vi "_builtins_rename_label.vi"(8 "error in (no error)":errorcluster, 10 "Label":string, 11 "GObject in":refnum<vi>) -> (0 "error out":errorcluster, 2 "has label?":bool, 3 "GObject out":refnum<vi>)   [LabVIEW 2019, in "Script.lvlib"]
doc: "Renames the GObject label if exists and moves the label to the appropriate position. If the label is empty this does nothing.\n\nCreated by: Ryan Pacini"
uses:
  _builtins_label_position.ctl
  Script.lvlib
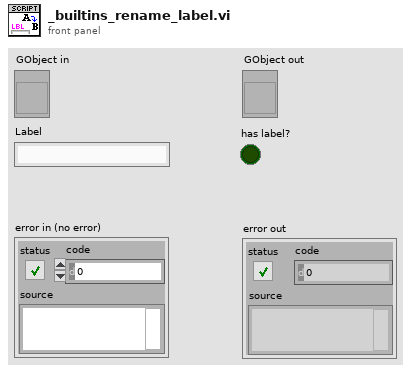
[diagram p1: front panel]
types:
  T1 = typedef "Script.lvlib/_builtins_label_position.ctl" = enum8{"Unchanged", "Top-left", "Top-middle", "Top-right", "Right-top", "Right-middle", "Right-bottom", "Bottom-right", "Bottom-middle", "Bottom-left", "Left-bottom", "Left-middle", "Left-top"}
  T2 = typedef "LVRectTypeDef.ctl" = cluster{"Left":i16, "Top":i16, "Right":i16, "Bottom":i16}
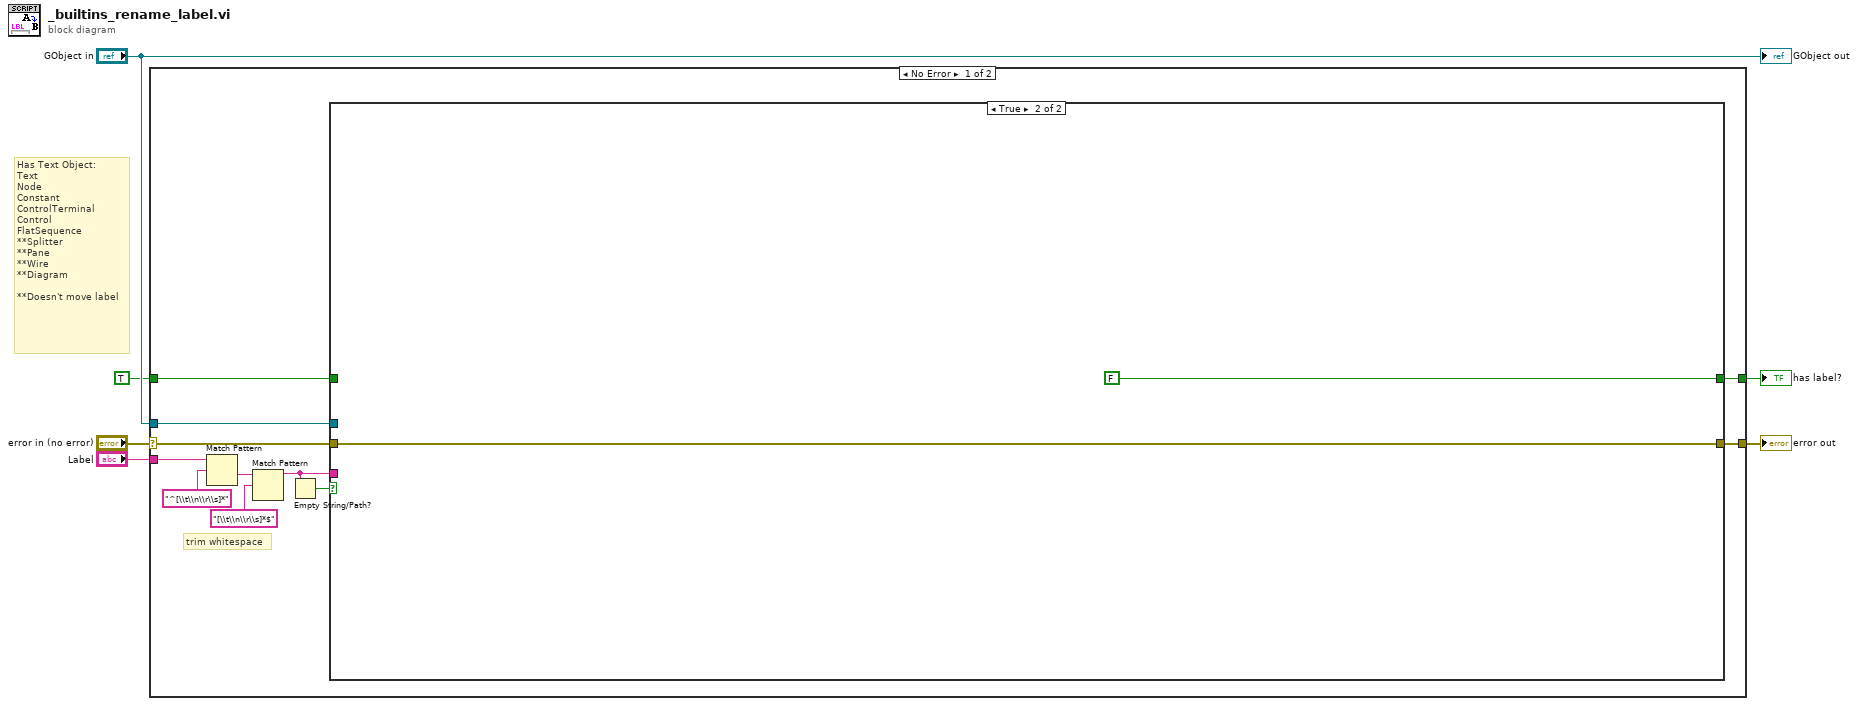
[diagram p0: block diagram]
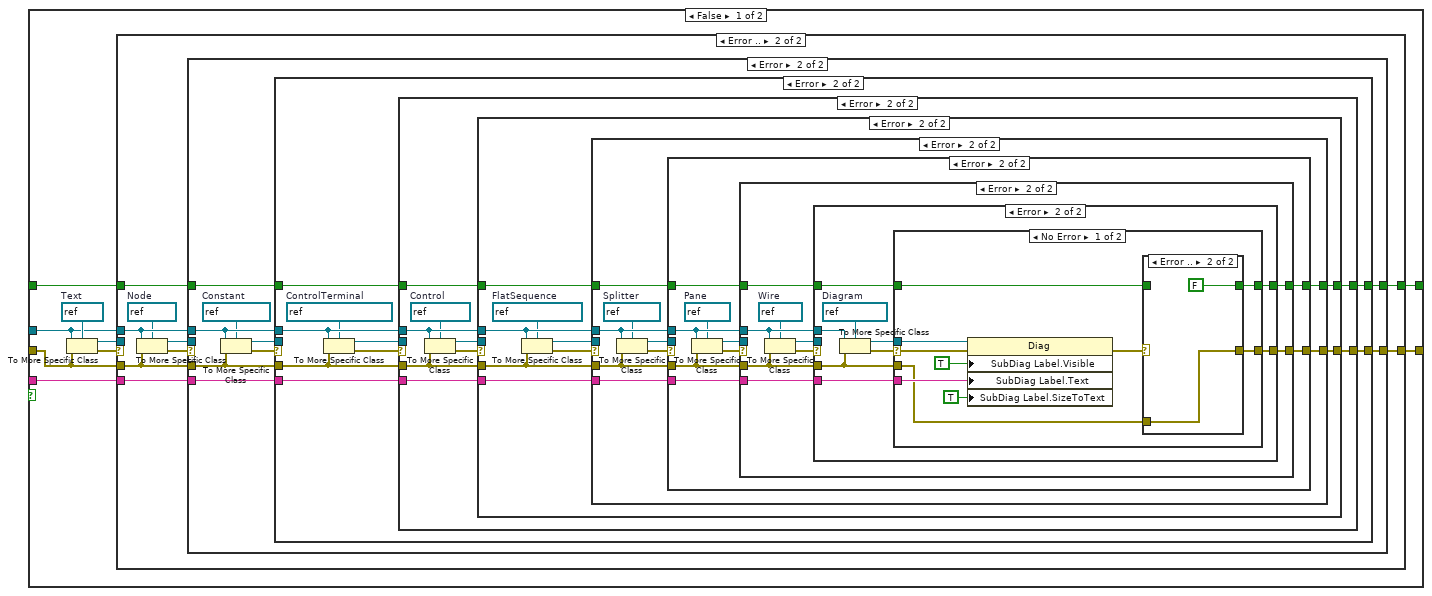
[diagram p2: hidden frame]
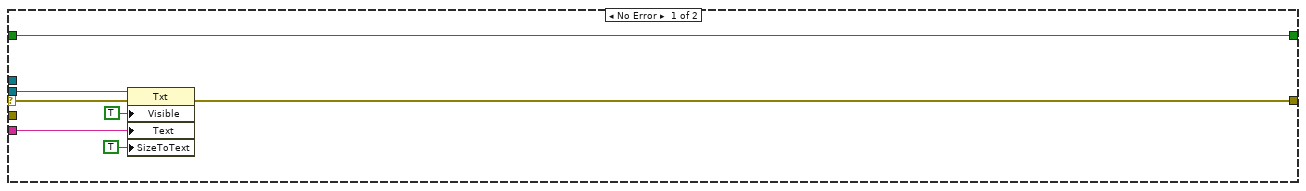
[diagram p3: hidden frame]
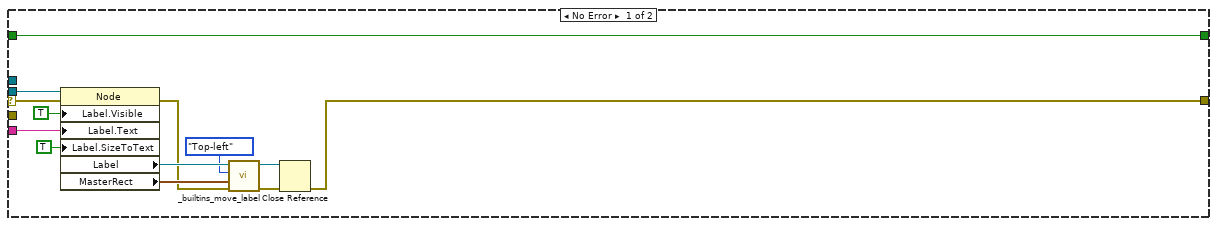
[diagram p4: hidden frame]
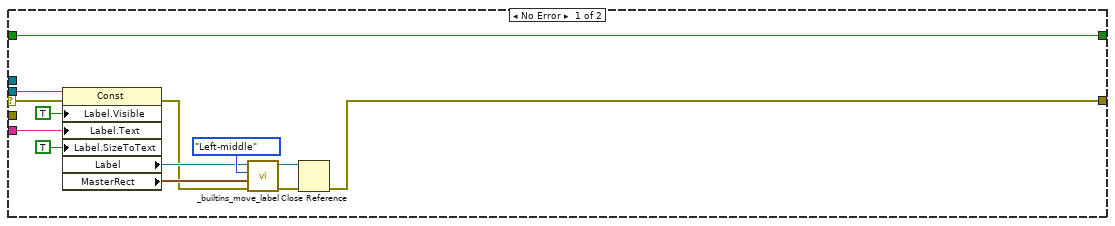
[diagram p5: hidden frame]
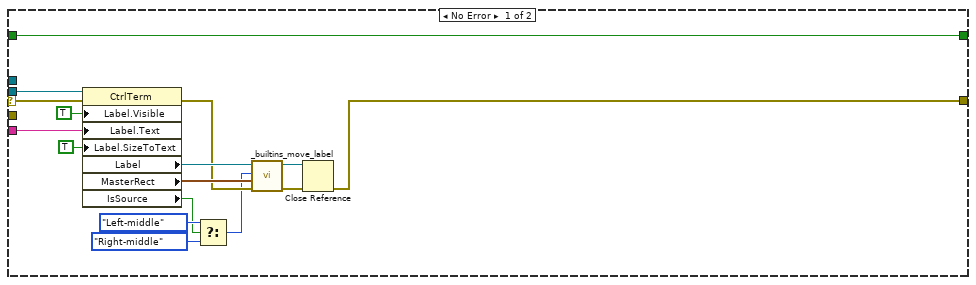
[diagram p6: hidden frame]
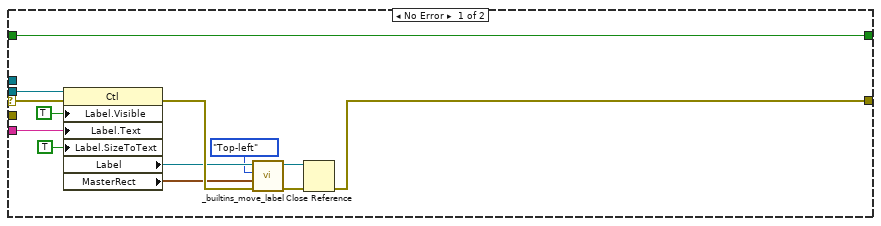
[diagram p7: hidden frame]
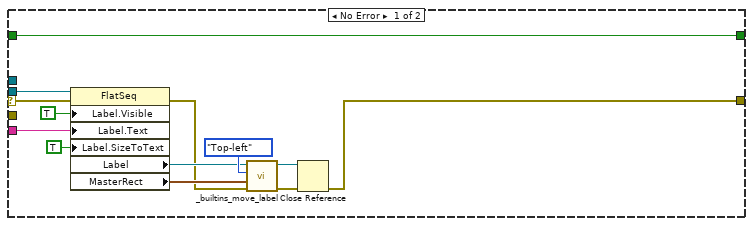
[diagram p8: hidden frame]
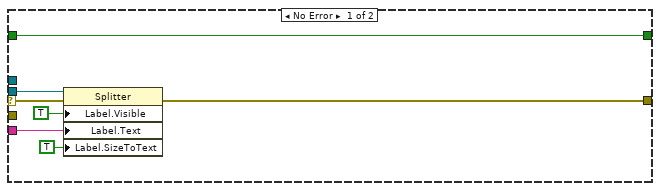
[diagram p9: hidden frame]
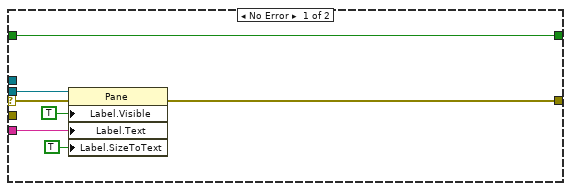
[diagram p10: hidden frame]
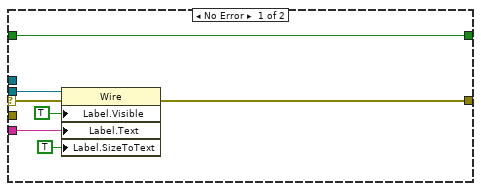
[diagram p11: hidden frame]
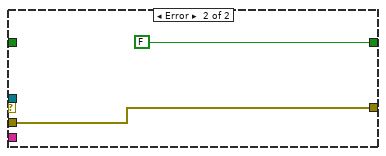
[diagram p13: hidden frame]
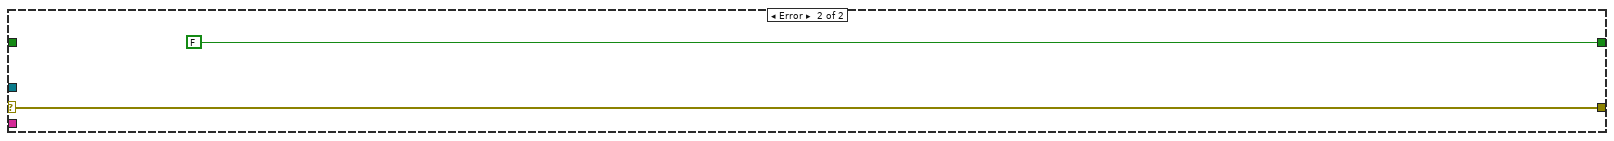
[diagram p14: hidden frame]
diagram:
  # "Has Text Object:\nText\nNode\nConstant\nControlTerminal\nControl\nFlatSequence\n**Splitter\n**Pane\n**Wire\n**Diagram\n\n**Doesn't move label"
  n1 = case shown="No Error" "error in (no error)" {
    selector: "error in (no error)" -> [w14 w223]
    tunnel: "GObject in" -> [w13 _]
    tunnel: [w17 w223] -> w2
    tunnel: [w16 FALSE] -> w3
    tunnel: "Label" -> [w9 _]
    tunnel: TRUE -> [w15 _]
    frame No Error {
      # "trim whitespace"
      n2 = Match Pattern(string=w9, regular expression="^[\\t\\n\\r\\s]*") -> (after substring=w12:string)  [unwired: 1 in, 3 out]
      n3 = Match Pattern(string=w12, regular expression="[\\t\\n\\r\\s]*$") -> (before substring=w8:string)  [unwired: 1 in, 3 out]
      n4 = Empty String/Path?(string/path=w8) -> (empty?=w7:bool)
      n5 = case shown="True" w7 {
        tunnel: [w26 w220] -> w17
        tunnel: [w25 FALSE] -> w16
        tunnel: w8 -> [w24 _]
        tunnel: w15 -> [w23 _]
        tunnel: w14 -> [w21 w220]
        tunnel: w13 -> [w20 _]
        frame False {
          w22 = refnum<vi> refnum  # Text
          n6 = To More Specific Class(target class=w22, reference=w20, error in=w21) -> (specific class reference=w18:refnum<vi>, error out=w19:errorcluster)
          n7 = case shown="Error .." w19 {
            selector: w19 -> [w32 _]
            tunnel: [w29 w42] -> w26
            tunnel: [w28 w41] -> w25
            tunnel: w21 -> [_ w38]
            tunnel: w20 -> [_ w37]
            tunnel: w24 -> [w31 w35]
            tunnel: w23 -> [w28 w34]
            tunnel: w18 -> [w33 _]
            frame No Error {
              n8 = property class="Txt"(reference=w33, error in=w32, "Visible"=TRUE, "Text"=w31, "SizeToText"=TRUE ("Size to Text?")) -> (error out=w29:errorcluster)  [unwired: 1 out]
            }
            frame Error {
              w36 = refnum<vi> refnum  # Node
              n9 = To More Specific Class(target class=w36, reference=w37, error in=w38) -> (specific class reference=w39:refnum<vi>, error out=w40:errorcluster)
              n10 = case shown="Error" w40 {
                selector: w40 -> [w55 _]
                tunnel: w37 -> [_ w62]
                tunnel: w39 -> [w54 _]
                tunnel: w38 -> [_ w61]
                tunnel: [w51 w60] -> w41
                tunnel: [w44 w59] -> w42
                tunnel: w35 -> [w52 w57]
                tunnel: w34 -> [w51 w56]
                frame No Error {
                  n11 = property class="Node"(reference=w54, error in=w55, "Label.Visible"=TRUE, "Label.Text"=w52, "Label.SizeToText"=TRUE ("Label.Size to Text?")) -> (error out=w45:errorcluster, "Label"=w50:refnum<vi>, "MasterRect"=w49:T2)  [unwired: 1 out]
                  n12 = call "_builtins_move_label.vi"("error in (no error)"=w45, "Owner Master Bounds Rect"=w49, "Label Position"=_builtins_label_position."Top-left", "Label in"=w50) -> ("error out"=w48:errorcluster, "dup Label"=w47:refnum<vi>)  [unwired: 6 in]
                  n13 = Close Reference(reference=w47, error in (no error)=w48) -> (error out=w44:errorcluster)
                }
                frame Error {
                  w58 = refnum<vi> refnum  # Constant
                  n14 = To More Specific Class(target class=w58, reference=w62, error in=w61) -> (specific class reference=w63:refnum<vi>, error out=w64:errorcluster)
                  n15 = case shown="Error" w64 {
                    selector: w64 -> [w77 _]
                    tunnel: w63 -> [w76 _]
                    tunnel: w62 -> [_ w84]
                    tunnel: w61 -> [_ w83]
                    tunnel: [w73 w81] -> w60
                    tunnel: [w66 w82] -> w59
                    tunnel: w57 -> [w75 w79]
                    tunnel: w56 -> [w73 w78]
                    frame No Error {
                      n16 = property class="Const"(reference=w76, error in=w77, "Label.Visible"=TRUE, "Label.Text"=w75, "Label.SizeToText"=TRUE ("Label.Size to Text?")) -> (error out=w67:errorcluster, "Label"=w69:refnum<vi>, "MasterRect"=w68:T2)  [unwired: 1 out]
                      n17 = call "_builtins_move_label.vi"("error in (no error)"=w67, "Owner Master Bounds Rect"=w68, "Label Position"=_builtins_label_position."Left-middle", "Label in"=w69) -> ("error out"=w72:errorcluster, "dup Label"=w71:refnum<vi>)  [unwired: 6 in]
                      n18 = Close Reference(reference=w71, error in (no error)=w72) -> (error out=w66:errorcluster)
                    }
                    frame Error {
                      w80 = refnum<vi> refnum  # ControlTerminal
                      n19 = To More Specific Class(target class=w80, reference=w84, error in=w83) -> (specific class reference=w85:refnum<vi>, error out=w86:errorcluster)
                      n20 = case shown="Error" w86 {
                        selector: w86 -> [w102 _]
                        tunnel: w85 -> [w101 _]
                        tunnel: w84 -> [_ w109]
                        tunnel: w83 -> [_ w108]
                        tunnel: [w92 w107] -> w82
                        tunnel: [w98 w106] -> w81
                        tunnel: w79 -> [w100 w104]
                        tunnel: w78 -> [w98 w103]
                        frame No Error {
                          n21 = property class="CtrlTerm"(reference=w101, error in=w102, "Label.Visible"=TRUE, "Label.Text"=w100, "Label.SizeToText"=TRUE ("Label.Size to Text?")) -> (error out=w93:errorcluster, "Label"=w95:refnum<vi>, "MasterRect"=w94:T2, "IsSource"=w89:bool)  [unwired: 1 out]
                          n22 = Select(t=_builtins_label_position."Left-middle" ("Label Position"), s=w89, f=_builtins_label_position."Right-middle" ("Label Position")) -> (s? t:f=w88:T1)
                          n23 = call "_builtins_move_label.vi"("error in (no error)"=w93, "Owner Master Bounds Rect"=w94, "Label Position"=w88, "Label in"=w95) -> ("error out"=w97:errorcluster, "dup Label"=w96:refnum<vi>)  [unwired: 6 in]
                          n24 = Close Reference(reference=w96, error in (no error)=w97) -> (error out=w92:errorcluster)
                        }
                        frame Error {
                          w105 = refnum<vi> refnum  # Control
                          n25 = To More Specific Class(target class=w105, reference=w109, error in=w108) -> (specific class reference=w110:refnum<vi>, error out=w111:errorcluster)
                          n26 = case shown="Error" w111 {
                            selector: w111 -> [w124 _]
                            tunnel: w110 -> [w123 _]
                            tunnel: w109 -> [_ w128]
                            tunnel: w108 -> [_ w131]
                            tunnel: [w116 w129] -> w107
                            tunnel: [w120 w130] -> w106
                            tunnel: w104 -> [w122 w126]
                            tunnel: w103 -> [w120 w125]
                            frame No Error {
                              n27 = property class="Ctl"(reference=w123, error in=w124, "Label.Visible"=TRUE, "Label.Text"=w122, "Label.SizeToText"=TRUE ("Label.Size to Text?")) -> (error out=w117:errorcluster, "Label"=w115:refnum<vi>, "MasterRect"=w114:T2)  [unwired: 1 out]
                              n28 = call "_builtins_move_label.vi"("error in (no error)"=w117, "Owner Master Bounds Rect"=w114, "Label Position"=_builtins_label_position."Top-left", "Label in"=w115) -> ("error out"=w119:errorcluster, "dup Label"=w118:refnum<vi>)  [unwired: 6 in]
                              n29 = Close Reference(reference=w118, error in (no error)=w119) -> (error out=w116:errorcluster)
                            }
                            frame Error {
                              w127 = refnum<vi> refnum  # FlatSequence
                              n30 = To More Specific Class(target class=w127, reference=w128, error in=w131) -> (specific class reference=w132:refnum<vi>, error out=w133:errorcluster)
                              n31 = case shown="Error" w133 {
                                selector: w133 -> [w146 _]
                                tunnel: w132 -> [w145 _]
                                tunnel: w131 -> [_ w153]
                                tunnel: [w142 w150] -> w130
                                tunnel: [w135 w151] -> w129
                                tunnel: w128 -> [_ w154]
                                tunnel: w126 -> [w144 w148]
                                tunnel: w125 -> [w142 w147]
                                frame No Error {
                                n32 = property class="FlatSeq"(reference=w145, error in=w146, "Label.Visible"=TRUE, "Label.Text"=w144, "Label.SizeToText"=TRUE ("Label.Size to Text?")) -> (error out=w136:errorcluster, "Label"=w138:refnum<vi>, "MasterRect"=w137:T2)  [unwired: 1 out]
                                n33 = call "_builtins_move_label.vi"("error in (no error)"=w136, "Owner Master Bounds Rect"=w137, "Label Position"=_builtins_label_position."Top-left", "Label in"=w138) -> ("error out"=w141:errorcluster, "dup Label"=w140:refnum<vi>)  [unwired: 6 in]
                                n34 = Close Reference(reference=w140, error in (no error)=w141) -> (error out=w135:errorcluster)
                                }
                                frame Error {
                                w149 = refnum<vi> refnum  # Splitter
                                n35 = To More Specific Class(target class=w149, reference=w154, error in=w153) -> (specific class reference=w152:refnum<vi>, error out=w155:errorcluster)
                                n36 = case shown="Error" w155 {
                                selector: w155 -> [w161 _]
                                tunnel: w154 -> [_ w166]
                                tunnel: w153 -> [_ w170]
                                tunnel: w152 -> [w162 _]
                                tunnel: [w157 w169] -> w151
                                tunnel: [w158 w168] -> w150
                                tunnel: w148 -> [w160 w164]
                                tunnel: w147 -> [w158 w163]
                                frame No Error {
                                n37 = property class="Splitter"(reference=w162, error in=w161, "Label.Visible"=TRUE, "Label.Text"=w160, "Label.SizeToText"=TRUE ("Label.Size to Text?")) -> (error out=w157:errorcluster)  [unwired: 1 out]
                                }
                                frame Error {
                                w165 = refnum<vi> refnum  # Pane
                                n38 = To More Specific Class(target class=w165, reference=w166, error in=w170) -> (specific class reference=w167:refnum<vi>, error out=w171:errorcluster)
                                n39 = case shown="Error" w171 {
                                selector: w171 -> [w178 _]
                                tunnel: w170 -> [_ w184]
                                tunnel: [w173 w183] -> w169
                                tunnel: [w174 w187] -> w168
                                tunnel: w167 -> [w177 _]
                                tunnel: w166 -> [_ w182]
                                tunnel: w164 -> [w175 w180]
                                tunnel: w163 -> [w174 w179]
                                frame No Error {
                                n40 = property class="Pane"(reference=w177, error in=w178, "Label.Visible"=TRUE, "Label.Text"=w175, "Label.SizeToText"=TRUE ("Label.Size to Text?")) -> (error out=w173:errorcluster)  [unwired: 1 out]
                                }
                                frame Error {
                                w181 = refnum<vi> refnum  # Wire
                                n41 = To More Specific Class(target class=w181, reference=w182, error in=w184) -> (specific class reference=w185:refnum<vi>, error out=w186:errorcluster)
                                n42 = case shown="Error" w186 {
                                selector: w186 -> [w193 _]
                                tunnel: [w190 w203] -> w187
                                tunnel: w185 -> [w194 _]
                                tunnel: w184 -> [_ w199]
                                tunnel: [w189 w198] -> w183
                                tunnel: w182 -> [_ w202]
                                tunnel: w180 -> [w192 w196]
                                tunnel: w179 -> [w190 w195]
                                frame No Error {
                                n43 = property class="Wire"(reference=w194, error in=w193, "Label.Visible"=TRUE, "Label.Text"=w192, "Label.SizeToText"=TRUE ("Label.Size to Text?")) -> (error out=w189:errorcluster)  [unwired: 1 out]
                                }
                                frame Error {
                                w197 = refnum<vi> refnum  # Diagram
                                n44 = To More Specific Class(target class=w197, reference=w202, error in=w199) -> (specific class reference=w200:refnum<vi>, error out=w201:errorcluster)
                                n45 = case shown="No Error" w201 {
                                selector: w201 -> [w209 _]
                                tunnel: [w210 FALSE] -> w203
                                tunnel: w200 -> [w213 _]
                                tunnel: w199 -> [w207 w218]
                                tunnel: [w211 w218] -> w198
                                tunnel: w196 -> [w208 _]
                                tunnel: w195 -> [w206 _]
                                frame No Error {
                                n46 = property class="Diag"(reference=w213, error in=w209, "SubDiag Label.Visible"=TRUE ("Subdiagram Label.Visible"), "SubDiag Label.Text"=w208, "SubDiag Label.SizeToText"=TRUE ("Subdiagram Label.Size to Text?")) -> (error out=w212:errorcluster)  [unwired: 1 out]
                                n47 = case shown="Error .." w212 {
                                selector: w212 -> [w215 _]
                                tunnel: [w215 w217] -> w211
                                tunnel: [w214 FALSE] -> w210
                                tunnel: w207 -> [_ w217]
                                tunnel: w206 -> [w214 _]
                                frame No Error {
                                }
                                frame Error {
                                }
                                }
                                }
                                frame Error {
                                }
                                }
                                }
                                }
                                }
                                }
                                }
                                }
                                }
                              }
                            }
                          }
                        }
                      }
                    }
                  }
                }
              }
            }
          }
        }
        frame True {
        }
      }
    }
    frame Error {
    }
  }
  "error out" <- w2
  "has label?" <- w3
  "GObject out" <- "GObject in"
